vi "FCI_Left_Cam_Coord.vi"(6 "Line Options":T3={"Number of Lines"=1, "Type"=enum."First Edge Rake", "Min. Score"=10.0, "Max. Score"=1000.0, "Orientation"=1.0, "Angle Range"=70.0, "Angle Tolerance"=1.0, "Step Size"=12, "Min. SNR (db)"=0.0, "Min. Points (%)"=25.0, "Hough Iterations"=5} {"Min. Points (%)" min=0.0 max=100.0; "Min. SNR (db)" min=0.0; "Max. Score" min=0.0 max=1024.0; "Min. Score" min=0.0 max=1024.0 step=1.0}, 7 "Edge Options":T5={"Edge Polarity"=2, "Kernel Size"=3, "Width"=3, "Minimum Edge Strength"=50.0, "Interpolation Type"=enum."Bilinear Fixed", "Data Processing Method"=enum."Average"} {"Edge Polarity" items=["All Edges", "Rising Edges", "Falling Edges"]; "Minimum Edge Strength" format="%.2f"; "Width" step=2; "Kernel Size" step=2}, 8 "error in (no error)":errorcluster, 9 "Search Direction":u32(ring)=2 items=["Left to Right", "Right to Left", "Top to Bottom", "Bottom to Top"], 10 "ROI":T1, 11 "Image Out":T7(plugin-control)) -> (0 "error out":errorcluster, 3 "Coordinate System":T2 {"Axis Reference" items=["Direct", "Indirect"]; "Angle (deg)" format="%.2f"; "Origin"."Y" format="%.2f"; "Origin"."X" format="%.2f"})   [LabVIEW 2019, in "Algorithm.lvclass"]
uses:
  FrameworkOverrides/Algorithm.lvclass
  <vilib>/vision/NI_Vision_Development_Module.lvlib
  <vilib>/vision/Measure.llb/Edge Polarity.ctl
  <vilib>/vision/Measure.llb/Edge Options.ctl
  <vilib>/vision/Measure.llb/Straight Edge Process.ctl
  <vilib>/vision/Measure.llb/Straight Edge Options.ctl
panel:
  out "Straightness 2":dbl
  out "Score 2":dbl
  out "Angle (Pixel) 2":dbl
  out "Straightness":dbl
  out "Score":dbl
  out "Angle (Pixel)":dbl
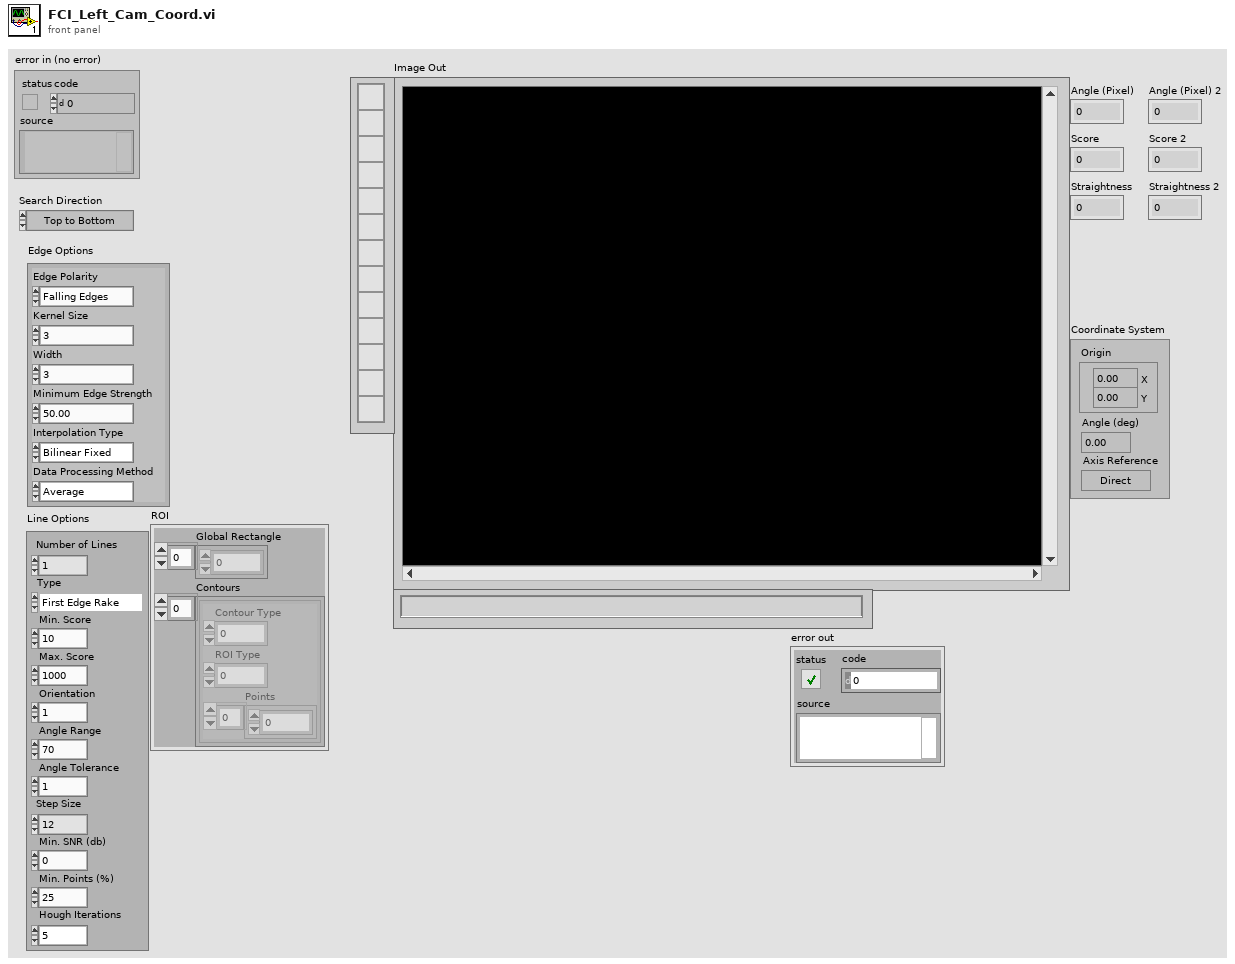
[diagram p1: front panel]
types:
  T1 = cluster{"Global Rectangle":i32[], "Contours":cluster{"Contour Type":u32, "ROI Type":u32, "Points":i32[]}[]}
  T2 = cluster{"Origin":cluster{"X":sgl, "Y":sgl}, "Angle (deg)":sgl, "Axis Reference":u32}
  T3 = typedef "Straight Edge Options.ctl" = cluster{"Number of Lines":i32, "Type":T4, "Min. Score":dbl, "Max. Score":dbl, "Orientation":dbl, "Angle Range":dbl, "Angle Tolerance":dbl, "Step Size":u32, "Min. SNR (db)":dbl, "Min. Points (%)":dbl, "Hough Iterations":i32}
  T4 = typedef "Straight Edge Process.ctl" = enum32{"First Edge Rake", "Best Edge Rake", "Hough Edge Rake", "First Edge Projection", "Best Edge Projection"}
  T5 = typedef "Edge Options.ctl" = cluster{"Edge Polarity":T6, "Kernel Size":u32, "Width":u32, "Minimum Edge Strength":sgl, "Interpolation Type":enum32{"Zero Order", "Bilinear", "Quadratic", "Cubic", "Bilinear Fixed"}, "Data Processing Method":enum32{"Average", "Median"}}
  T6 = typedef "Edge Polarity.ctl" = u32
  T7 = typedef "IMAQ Image.ctl" = refnum<image>
  T8 = cluster{"Point1 (Pixels)":cluster{"X":sgl, "Y":sgl}, "Point2 (Pixels)":cluster{"X":sgl, "Y":sgl}, "Point1 (Real-World)":cluster{"X":sgl, "Y":sgl}, "Point2 (Real-World)":cluster{"X":sgl, "Y":sgl}, "Angle (Pixel)":dbl, "Angle (Real-World)":dbl, "Score":dbl, "Straightness":dbl, "Average SNR (db)":dbl, "Calibration Valid":bool}[]
  T9 = typedef "Search Line.ctl" = cluster{"Start Point":cluster{"X":sgl, "Y":sgl}, "End Point":cluster{"X":sgl, "Y":sgl}, "Edge Info":T10[], "Edge Map":dbl[], "Calibration Valid":bool}
  T10 = typedef "Edge New.ctl" = cluster{"Location (Pixel)":cluster{"X":sgl, "Y":sgl}, "Location (Real-World)":cluster{"X":sgl, "Y":sgl}, "Distance (Pixel)":dbl, "Distance (Real-World)":dbl, "Strength":dbl, "Noise":dbl, "Rising?":bool}
  T11 = cluster{"Point1 (Pixels)":cluster{"X":sgl, "Y":sgl}, "Point2 (Pixels)":cluster{"X":sgl, "Y":sgl}, "Point1 (Real-World)":cluster{"X":sgl, "Y":sgl}, "Point2 (Real-World)":cluster{"X":sgl, "Y":sgl}, "Angle (Pixel)":dbl, "Angle (Real-World)":dbl, "Score":dbl, "Straightness":dbl, "Average SNR (db)":dbl, "Calibration Valid":bool}
  T12 = cluster{"Point1 (Pixels)":cluster{"X":sgl, "Y":sgl}, "Point2 (Pixels)":cluster{"X":sgl, "Y":sgl}}
  T13 = cluster{"Intersection Point":cluster{"X":sgl, "Y":sgl}}
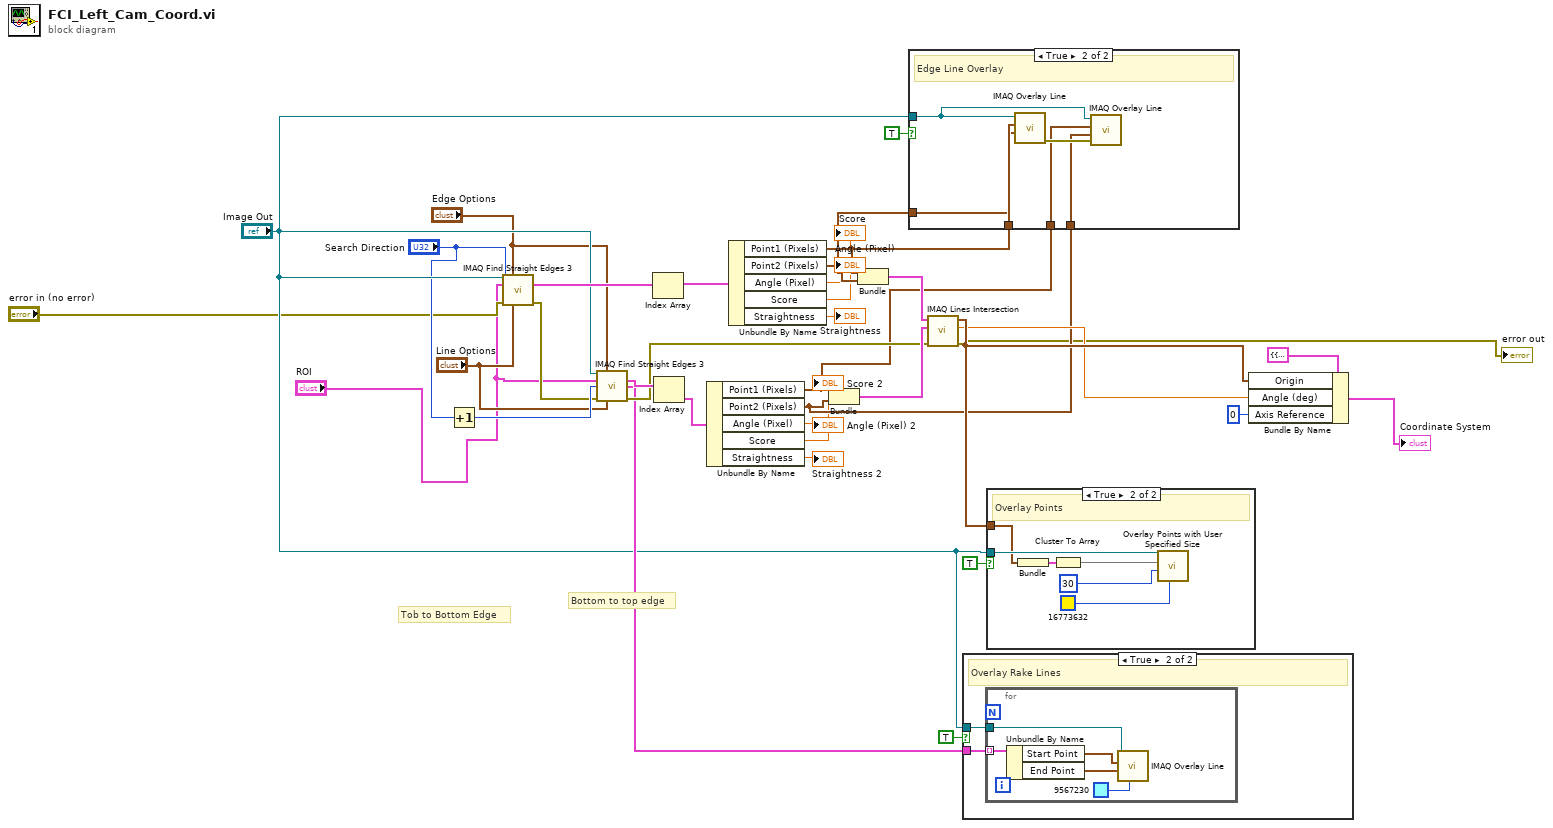
[diagram p0: block diagram]
diagram:
  # "Bottom to top edge"
  # "Tob to Bottom Edge"
  n1 = Increment(x="Search Direction") -> (x+1=w7:u32)
  n2 = call "IMAQ Find Straight Edges 3"("Image"="Image Out", "Edge Options"="Edge Options", "ROI Descriptor"="ROI", "Search Direction"="Search Direction", "error in (no error)"="error in (no error)", "Line Options"="Line Options") -> ("Straight Edges"=w35:T8, "error out"=w4:errorcluster)  [unwired: 5 in, 3 out]
  n3 = call "IMAQ Find Straight Edges 3"("Image"="Image Out", "Edge Options"="Edge Options", "ROI Descriptor"="ROI", "Search Direction"=w7, "error in (no error)"=w4, "Line Options"="Line Options") -> ("Straight Edges"=w33:T8, "Search Lines Information"=w18:T9[], "error out"=w29:errorcluster)  [unwired: 5 in, 2 out]
  n4 = Index Array(array=w35) -> (element=w34:T11)  [unwired: 1 in]
  n5 = Index Array(array=w33) -> (element=w32:T11)  [unwired: 1 in]
  n6 = Unbundle By Name(w32) -> ("Point1 (Pixels)"=w22:cluster{"X":sgl, "Y":sgl}, "Point2 (Pixels)"=w21:cluster{"X":sgl, "Y":sgl}, "Angle (Pixel)"=→"Angle (Pixel) 2":dbl, "Score"=→"Score 2":dbl, "Straightness"=→"Straightness 2":dbl)
  n7 = Unbundle By Name(w34) -> ("Point1 (Pixels)"=w24:cluster{"X":sgl, "Y":sgl}, "Point2 (Pixels)"=w23:cluster{"X":sgl, "Y":sgl}, "Angle (Pixel)"=→"Angle (Pixel)":dbl, "Score"=→"Score":dbl, "Straightness"=→"Straightness":dbl)
  n8 = Bundle("Point1 (Pixels)"=w22, "Point2 (Pixels)"=w21) -> (w30:T12)  [unwired: 1 in]
  n9 = Bundle("Point1 (Pixels)"=w24, "Point2 (Pixels)"=w23) -> (w31:T12)  [unwired: 1 in]
  n10 = case shown="True" TRUE {
    tunnel: "Image Out" -> [_ w36]
    tunnel: w24 -> [_ w40]
    tunnel: w23 -> [_ w39]
    tunnel: w22 -> [_ w38]
    tunnel: w21 -> [_ w37]
    frame False {
    }
    frame True {
      # "Edge Line Overlay"
      n11 = call "IMAQ Overlay Line"("End Point"=w39, "Start Point"=w40, "Image"=w36) -> ("error out"=w41:errorcluster)  [unwired: 7 in, 1 out]
      n12 = call "IMAQ Overlay Line"("error in (no error)"=w41, "End Point"=w37, "Start Point"=w38, "Image"=w36) -> ()  [unwired: 6 in, 2 out]
    }
  }
  n13 = call "IMAQ Lines Intersection"("error in (no error)"=w29, "Line 2"=w30, "Line 1"=w31) -> ("error out"=→"error out":errorcluster, "Angle"=w26:dbl, "Intersection Point"=w27:cluster{"X":sgl, "Y":sgl})  [unwired: 6 in]
  n14 = case shown="True" TRUE {
    tunnel: w18 -> [_ w43]
    tunnel: "Image Out" -> [_ w42]
    frame False {
    }
    frame True {
      # "Overlay Rake Lines"
      n15 = for {
        tunnel: w43 -> [w48] mode=indexing
        tunnel: w42 -> [w45]
        n16 = Unbundle By Name(w48) -> ("Start Point"=w47:cluster{"X":sgl, "Y":sgl}, "End Point"=w46:cluster{"X":sgl, "Y":sgl})
        n17 = call "IMAQ Overlay Line"("Color"=u32 9567230, "End Point"=w46, "Start Point"=w47, "Image"=w45) -> ()  [unwired: 6 in, 2 out]
      }
    }
  }
  n18 = case shown="True" TRUE {
    tunnel: w27 -> [_ w51]
    tunnel: "Image Out" -> [_ w54]
    frame False {
    }
    frame True {
      # "Overlay Points"
      n19 = Bundle("Intersection Point"=w51) -> (w50:T13)  [unwired: 1 in]
      n20 = Cluster To Array(cluster=w50) -> (array=w49:cluster{"X":sgl, "Y":sgl}[])
      n21 = call "Overlay Points with User Specified Size.vi"("Color"=u32 16773632, "Point Diameter (5)"=u32 30, "Points"=w49, "Image In"=w54) -> ()  [unwired: 6 in, 2 out]
    }
  }
  n22 = Bundle By Name(cluster=T2 {"Origin"={"X"=0.0, "Y"=0.0}, "Angle (deg)"=0.0, "Axis Reference"=0} ("Coordinate System"), "Origin"=w27, "Angle (deg)"=w26, "Axis Reference"=u32 0) -> (→"Coordinate System":T2)
